vi "Board Calibrator.vi"(7 "Board":T1 items=["Quad DC Board", "Lens 1 (Slot 8) Module", "Lens 2 (Slot 6) Module", "Detector Board", "Quad DC Board with Test Points", "Lens 1 Module with Test Points", "Len 2 Module with Test Points", "", "", "", "", "", "", "", ""]) -> (2 "ADC Table":T2[](array[typedef]), 3 "Suceeded":bool)   [LabVIEW 2018]
uses:
  Type/_RT Configuration 2.ctl
  Type/_Board ID.ctl
  Type/_Model Family.ctl
  Type/_RT Command.ctl
  <vilib>/printing/EasyPrintingControls.llb/layout_options.ctl
  <vilib>/printing/EasyPrintingControls.llb/orientation.ctl
  <vilib>/printing/EasyPrintingControls.llb/panel_scaling_for_page.ctl
  <vilib>/printing/EasyPrintingControls.llb/margins.ctl
  <vilib>/printing/EasyPrintingControls.llb/margin_values.ctl
  <vilib>/printing/EasyPrintingControls.llb/measurement_system.ctl
  <vilib>/printing/EasyPrintingControls.llb/printer_options.ctl
  <vilib>/printing/EasyPrintingControls.llb/printing_method.ctl
  <vilib>/printing/EasyPrintingControls.llb/color_or_monochrome.ctl
  <vilib>/printing/EasyPrintingControls.llb/page_header_options.ctl
  <vilib>/printing/EasyPrintingControls.llb/page_headers.ctl
  <vilib>/printing/EasyPrintingControls.llb/page_header_content_options.ctl
  <vilib>/printing/EasyPrinting.llb/Easy Print VI Panel or Documentation (path).vi
  <vilib>/Utility/NIReport.llb/NI_ReportGenerationCore.lvlib
panel:
  in  "Print":bool
  in  "ADC Channel Calibration":string[][](table)
  in  "Done":bool
  in  "Start":bool
  in  "DAC Channel Calibration":string[][](table)
  out "Current Task":string="Press Start Calibration button to begin or Done button to exit"
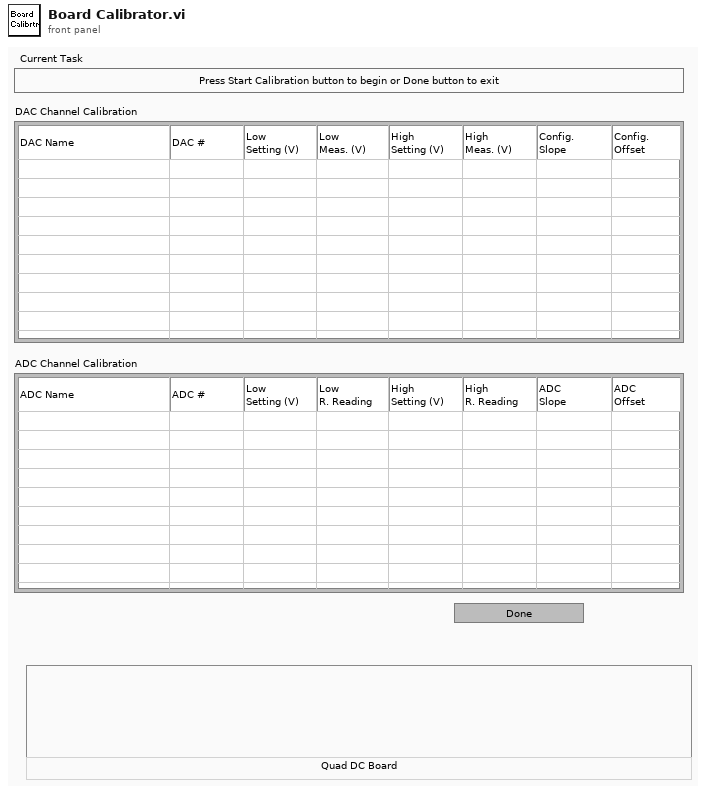
[diagram p1: front panel]
types:
  T1 = typedef "_Board ID.ctl" = u16
  T2 = typedef "_RT Configuration 2.ctl" = cluster{"Name":string, "Ch#":u8, "Min":dbl, "Max":dbl, "Def+":dbl, "Def-":dbl, "Offset":dbl, "Slope":dbl, "Type":u8, "Description":string, "SettleT":dbl}
  T3 = typedef "_RT Command.ctl" = enum16{"xml Start Run", "xml Start Actual Run", "xml Stop Run", "xml Runtime Update", "xml Get Status", "xml Get Table", "xml Set Table", "xml Get Configuration", "xml System Status", "xml Set LC Input Logic", "xml Get Data", "xml Get Info", "Start", "StartActualRun", "Stop", "Runtime Update", "Get Data", "Get Info", "Get Status", "Get Param", "Get Config", "Get Table", "Read ADC", "Set Oscillator", "Update Config", "Update Table", "Set All Pol", "Set Pol and DC", "Set Max Mass", "Toggle RP", "Toggle EL", "Set PIC", "Initialize Turbo", "Send Turbo Comm", "Close Turbo", "P1", "P2", "P3", "Send Serial", "Set LC Out", "Get LC In", "Read VAC", "Test Table", "Toggle Power", "Get Startup", "Set Startup", "Get ADC Table", "Set ADC Table", "Get Brief Status", "Get Detail Status", "Auxiliary Update", "Set CC Logics", "Test Channel", "Set CC Input Logics", "Ignore Error", "invalid"}
  T4 = typedef "NI_ReportGenerationCore.lvlib/layout_options.ctl" = cluster{"orientation (unchanged)":T5, "panel scaling for page (unchanged)":T6, "margins":T7, "printer options":T10, "page header options":T13}
  T5 = typedef "NI_ReportGenerationCore.lvlib/orientation.ctl" = u16
  T6 = typedef "NI_ReportGenerationCore.lvlib/panel_scaling_for_page.ctl" = u16
  T7 = typedef "NI_ReportGenerationCore.lvlib/margins.ctl" = cluster{"override VI margins (false)":bool, "margins (1.00)":T8, "measurement system (default)":T9}
  T8 = typedef "NI_ReportGenerationCore.lvlib/margin_values.ctl" = cluster{"top":dbl, "left":dbl, "right":dbl, "bottom":dbl}
  T9 = typedef "NI_ReportGenerationCore.lvlib/measurement_system.ctl" = u16
  T10 = typedef "NI_ReportGenerationCore.lvlib/printer_options.ctl" = cluster{"destination printer name (current)":string, "printing method (unchanged)":T11, "color or monochrome (unchanged)":T12}
  T11 = typedef "NI_ReportGenerationCore.lvlib/printing_method.ctl" = u16
  T12 = typedef "NI_ReportGenerationCore.lvlib/color_or_monochrome.ctl" = u16
  T13 = typedef "NI_ReportGenerationCore.lvlib/page_header_options.ctl" = cluster{"page headers (unchanged)":T14, "page header content options":T15}
  T14 = typedef "NI_ReportGenerationCore.lvlib/page_headers.ctl" = u16
  T15 = typedef "NI_ReportGenerationCore.lvlib/page_header_content_options.ctl" = cluster{"Include VI Name":bool, "Include VI Path":bool, "Include Last Modification Date":bool, "Include Date Printed":bool, "Include Page Number":bool, "Include VI Icon":bool}
  T16 = typedef "_Model Family.ctl" = u16
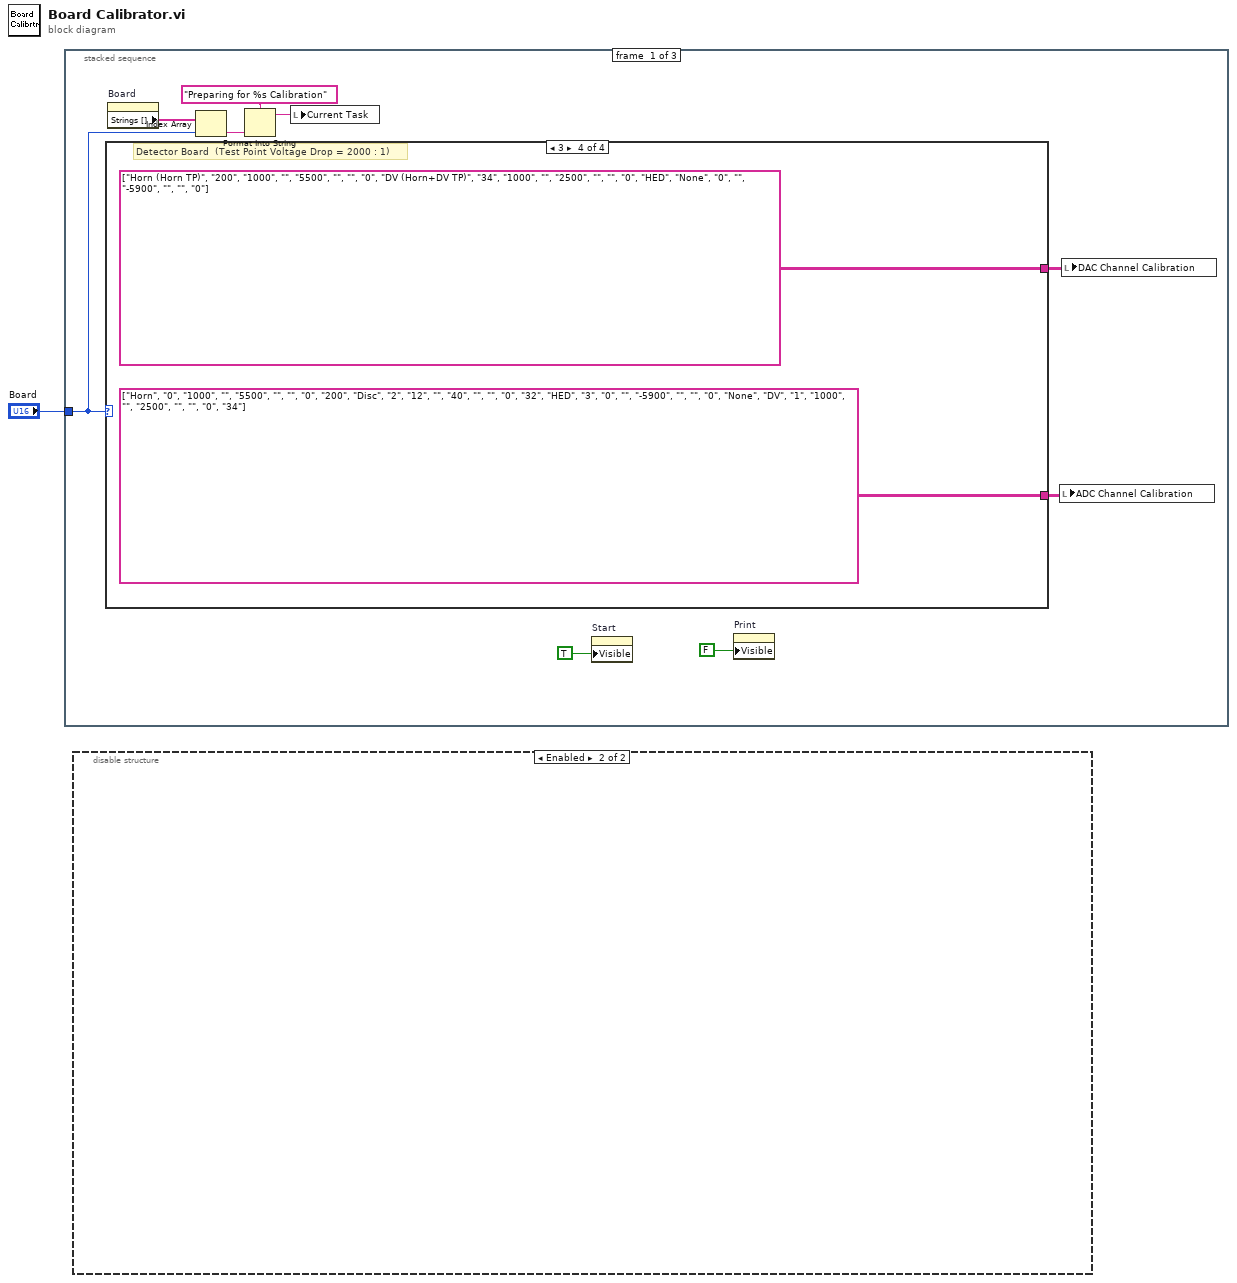
[diagram p0: block diagram]
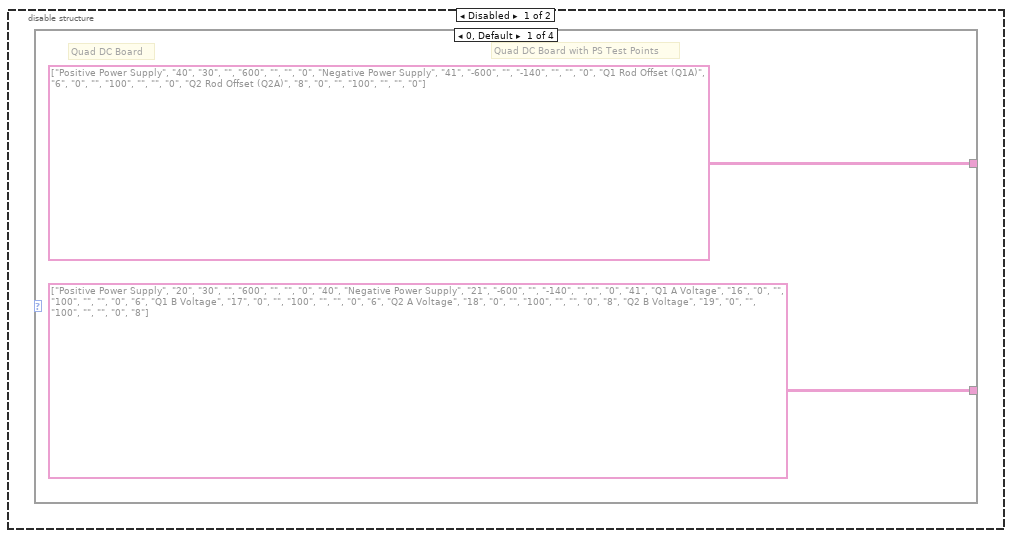
[diagram p2: hidden frame]
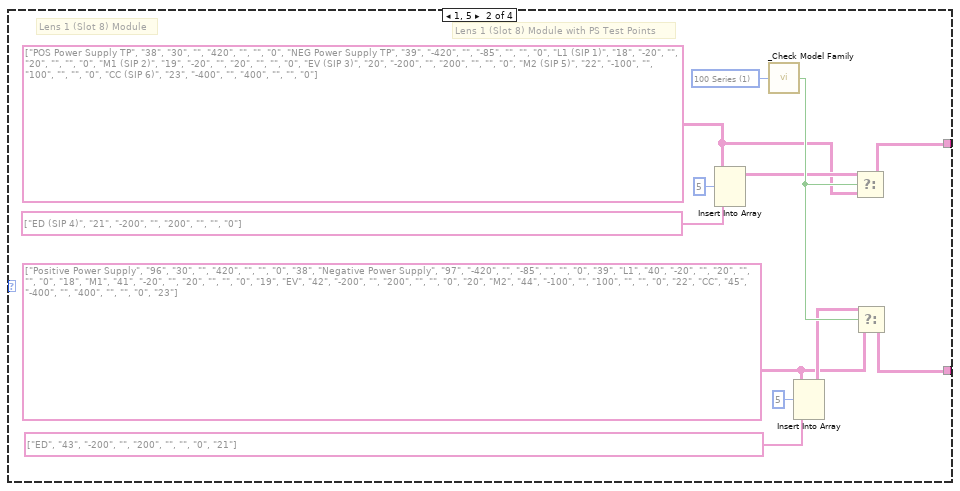
[diagram p3: hidden frame]
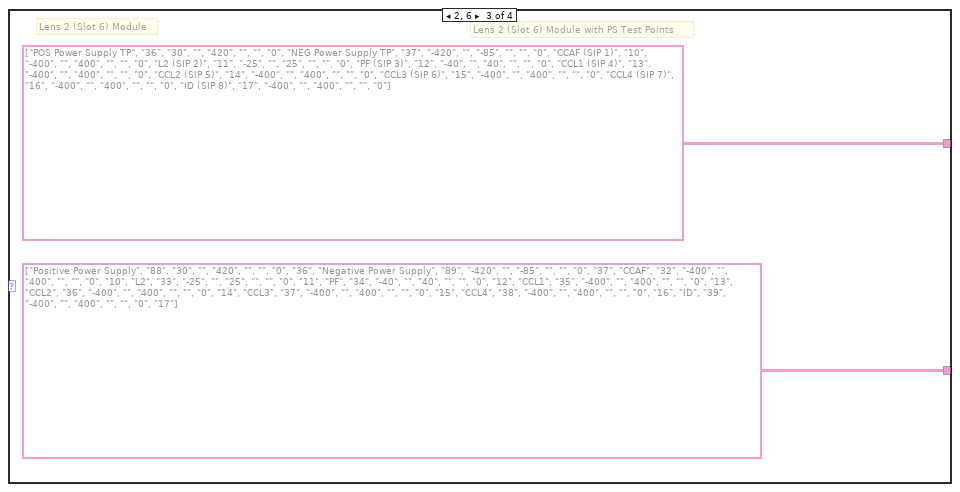
[diagram p4: hidden frame]
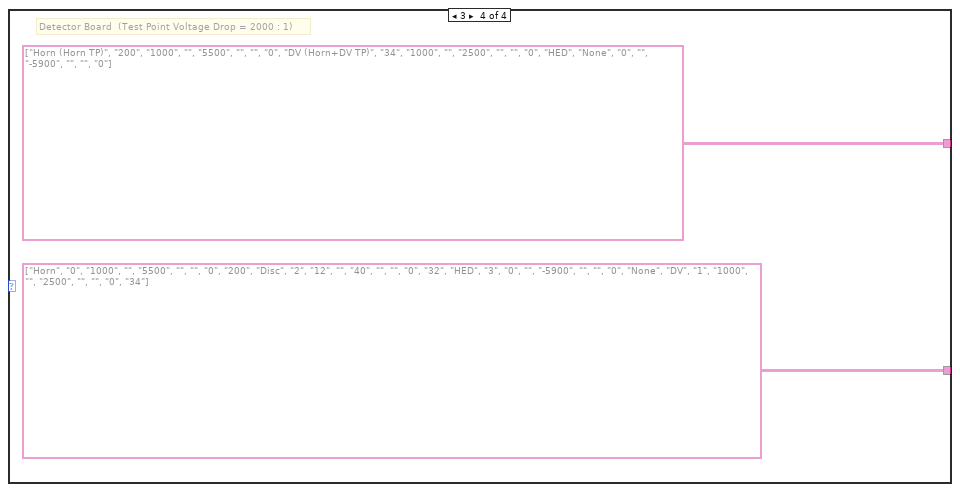
[diagram p5: hidden frame]
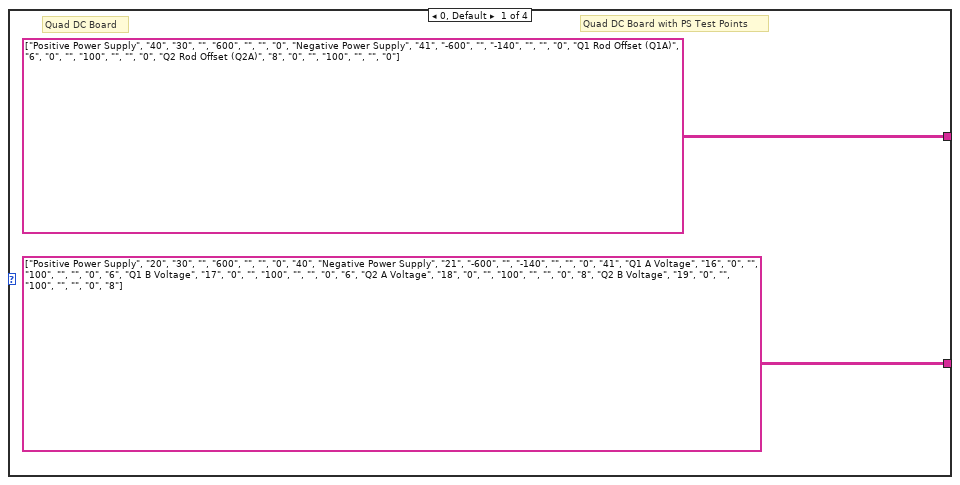
[diagram p6: hidden frame]
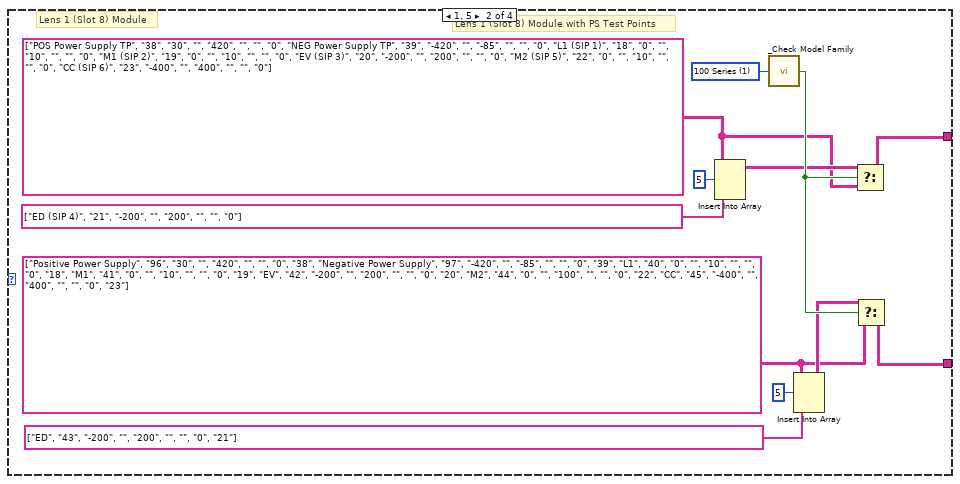
[diagram p7: hidden frame]
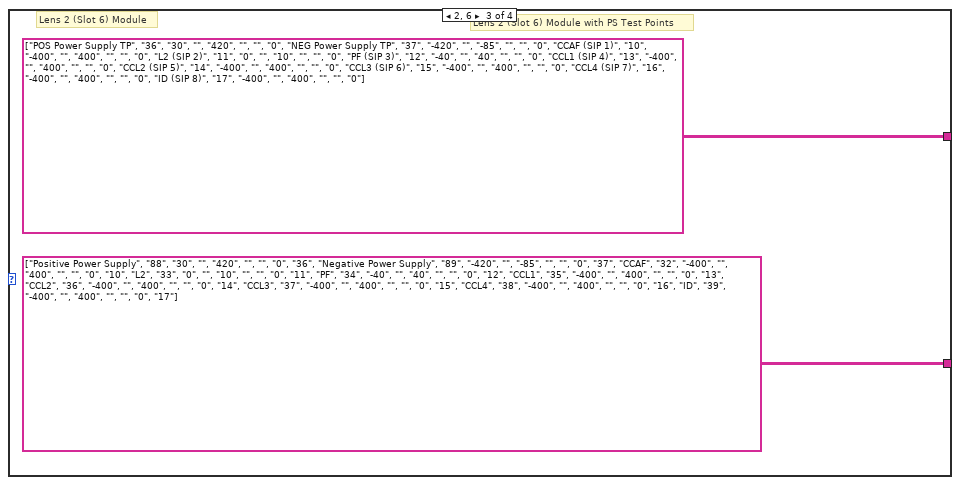
[diagram p8: hidden frame]
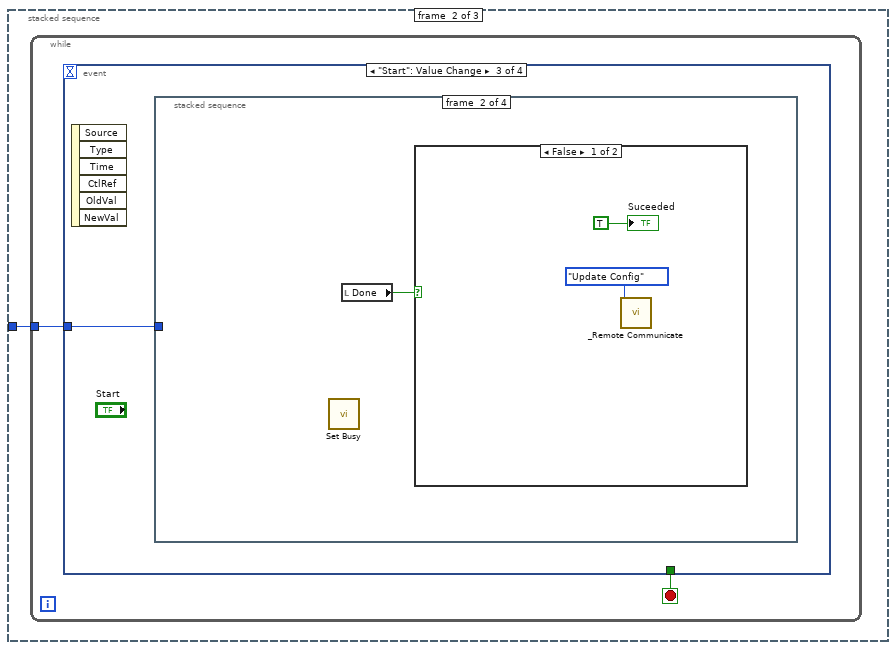
[diagram p9: hidden frame]
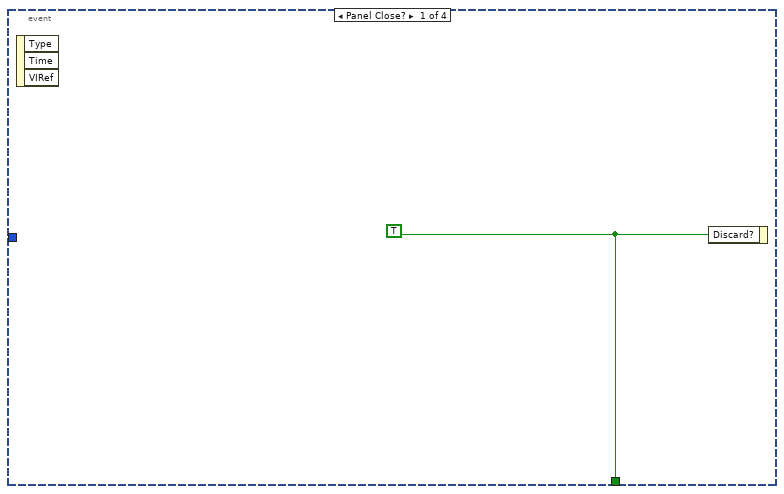
[diagram p10: hidden frame]
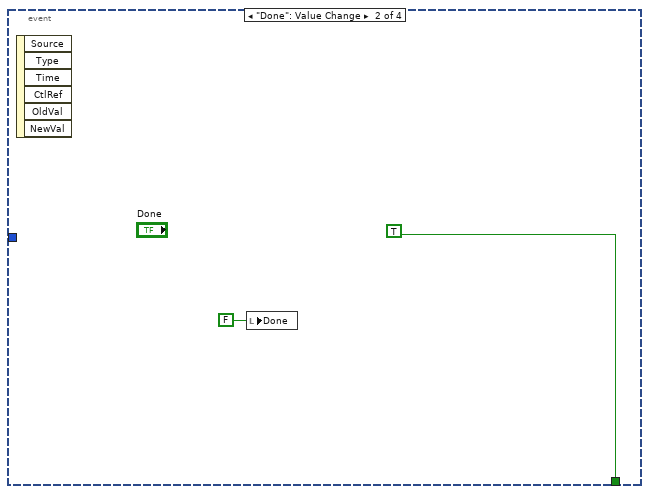
[diagram p11: hidden frame]
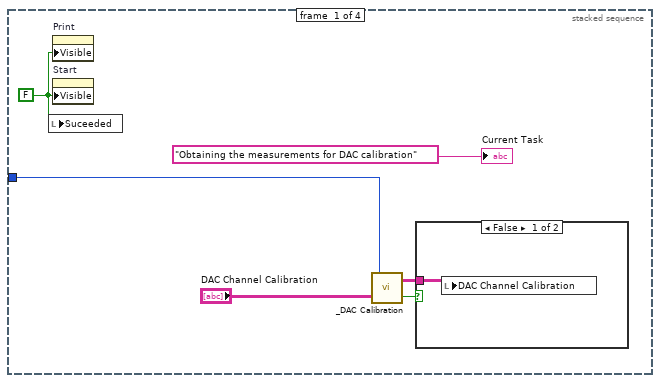
[diagram p12: hidden frame]
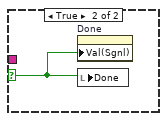
[diagram p13: hidden frame]
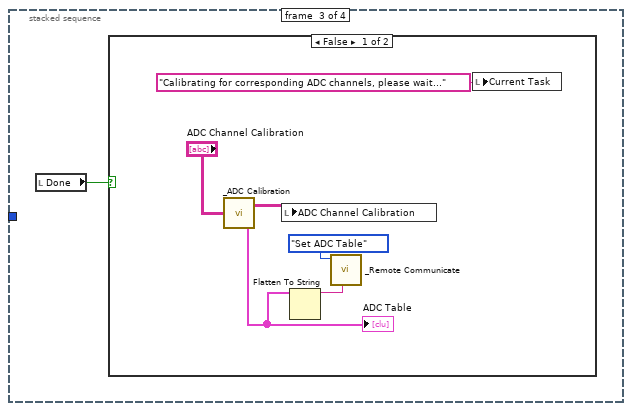
[diagram p15: hidden frame]
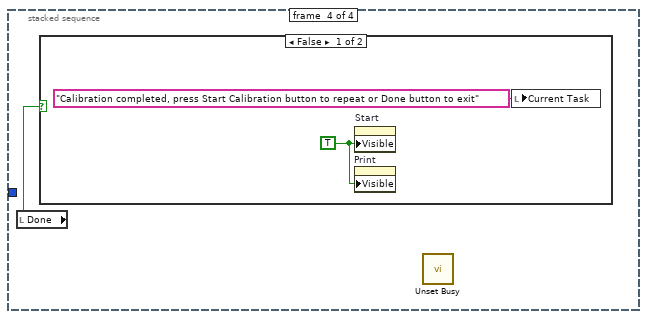
[diagram p17: hidden frame]
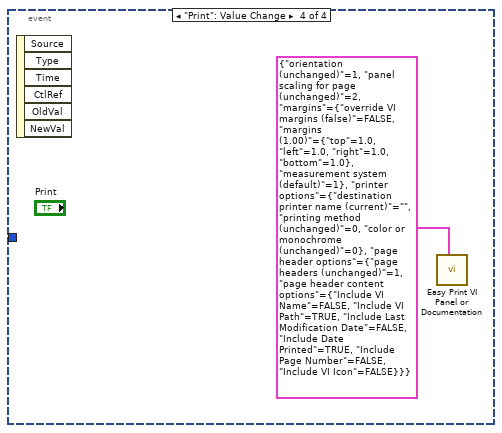
[diagram p19: hidden frame]
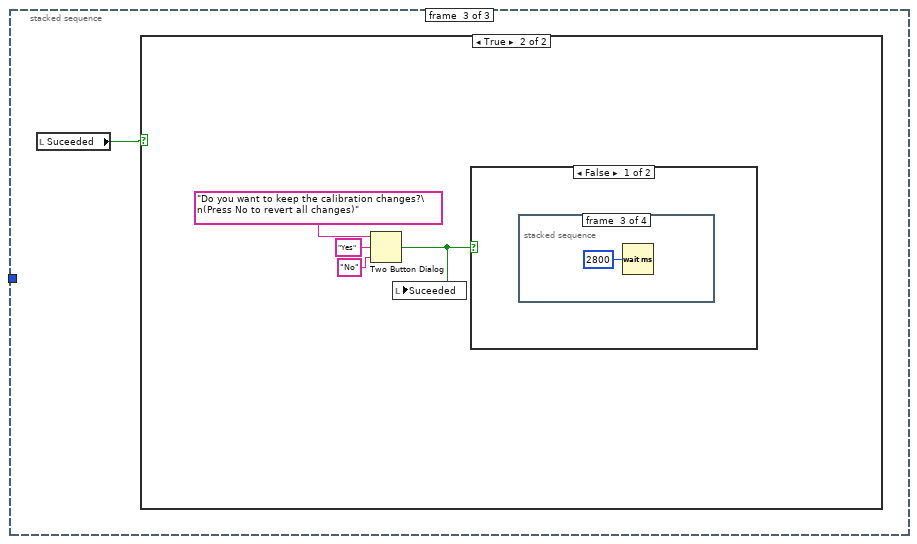
[diagram p20: hidden frame]
diagram:
  n1 = stacked-sequence {
    tunnel: "Board" -> [w6 w29 _]
    frame #0 {
      n2 = case shown="3" w6 {
        tunnel: [string[][] [["Positive Power Supply", "20", "30", "", "600", "", "", "0", "40"], ["Negative Power Supply", "21", "-600", "", "-140", "", "", "0", "41"], ["Q1 A Voltage", "16", "0", "", "100", "", "", "0", "6"], ["Q1 B Voltage", "17", "0", "", "100", "", "", "0", "6"], ["Q2 A Voltage", "18", "0", "", "100", "", "", "0", "8"], ["Q2 B Voltage", "19", "0", "", "100", "", "", "0", "8"]] ("ADC Channel Calibration") w13 string[][] [["Positive Power Supply", "88", "30", "", "420", "", "", "0", "36"], ["Negative Power Supply", "89", "-420", "", "-85", "", "", "0", "37"], ["CCAF", "32", "-400", "", "400", "", "", "0", "10"], ["L2", "33", "0", "", "10", "", "", "0", "11"], ["PF", "34", "-40", "", "40", "", "", "0", "12"], ["CCL1", "35", "-400", "", "400", "", "", "0", "13"], ["CCL2", "36", "-400", "", "400", "", "", "0", "14"], ["CCL3", "37", "-400", "", "400", "", "", "0", "15"], ["CCL4", "38", "-400", "", "400", "", "", "0", "16"], ["ID", "39", "-400", "", "400", "", "", "0", "17"]] ("ADC Channel Calibration") string[][] [["Horn", "0", "1000", "", "5500", "", "", "0", "200"], ["Disc", "2", "12", "", "40", "", "", "0", "32"], ["HED", "3", "0", "", "-5900", "", "", "0", "None"], ["DV", "1", "1000", "", "2500", "", "", "0", "34"]] ("ADC Channel Calibration")] -> w10
        tunnel: [string[][] [["Positive Power Supply", "40", "30", "", "600", "", "", "0"], ["Negative Power Supply", "41", "-600", "", "-140", "", "", "0"], ["Q1 Rod Offset (Q1A)", "6", "0", "", "100", "", "", "0"], ["Q2 Rod Offset (Q2A)", "8", "0", "", "100", "", "", "0"]] ("DAC Channel Calibration") w16 string[][] [["POS Power Supply TP", "36", "30", "", "420", "", "", "0"], ["NEG Power Supply TP", "37", "-420", "", "-85", "", "", "0"], ["CCAF (SIP 1)", "10", "-400", "", "400", "", "", "0"], ["L2 (SIP 2)", "11", "0", "", "10", "", "", "0"], ["PF (SIP 3)", "12", "-40", "", "40", "", "", "0"], ["CCL1 (SIP 4)", "13", "-400", "", "400", "", "", "0"], ["CCL2 (SIP 5)", "14", "-400", "", "400", "", "", "0"], ["CCL3 (SIP 6)", "15", "-400", "", "400", "", "", "0"], ["CCL4 (SIP 7)", "16", "-400", "", "400", "", "", "0"], ["ID (SIP 8)", "17", "-400", "", "400", "", "", "0"]] ("DAC Channel Calibration") string[][] [["Horn (Horn TP)", "200", "1000", "", "5500", "", "", "0"], ["DV (Horn+DV TP)", "34", "1000", "", "2500", "", "", "0"], ["HED", "None", "0", "", "-5900", "", "", "0"]] ("DAC Channel Calibration")] -> w9
        frame 0, Default {
          # "Quad DC Board with PS Test Points"
          # "Quad DC Board"
        }
        frame 1, 5 {
          w20 = T16 1 items=["8080 Series", "100 Series", "200 Series", "300 Series", "Other Series"] ("Model Family (100)")
          w14 = string[][] [["Positive Power Supply", "96", "30", "", "420", "", "", "0", "38"], ["Negative Power Supply", "97", "-420", "", "-85", "", "", "0", "39"], ["L1", "40", "0", "", "10", "", "", "0", "18"], ["M1", "41", "0", "", "10", "", "", "0", "19"], ["EV", "42", "-200", "", "200", "", "", "0", "20"], ["M2", "44", "0", "", "100", "", "", "0", "22"], ["CC", "45", "-400", "", "400", "", "", "0", "23"]] ("ADC Channel Calibration")
          w17 = string[][] [["POS Power Supply TP", "38", "30", "", "420", "", "", "0"], ["NEG Power Supply TP", "39", "-420", "", "-85", "", "", "0"], ["L1 (SIP 1)", "18", "0", "", "10", "", "", "0"], ["M1 (SIP 2)", "19", "0", "", "10", "", "", "0"], ["EV (SIP 3)", "20", "-200", "", "200", "", "", "0"], ["M2 (SIP 5)", "22", "0", "", "10", "", "", "0"], ["CC (SIP 6)", "23", "-400", "", "400", "", "", "0"]] ("DAC Channel Calibration")
          # "Lens 1 (Slot 8) Module with PS Test Points"
          # "Lens 1 (Slot 8) Module"
          n3 = Insert Into Array(array=w17, index (row)=5, new element=string[] ["ED (SIP 4)", "21", "-200", "", "200", "", "", "0"] ("new element/subarray")) -> (w18:string[][])  [unwired: 1 in]
          n4 = call "_Check Model Family.vi"("Model Family (100)"=w20) -> ("Yes"=w19:bool)
          n5 = Insert Into Array(array=w14, index (row)=5, new element=string[] ["ED", "43", "-200", "", "200", "", "", "0", "21"] ("new element/subarray")) -> (w15:string[][])  [unwired: 1 in]
          n6 = Select(t=w18, s=w19, f=w17) -> (s? t:f=w16:string[][])
          n7 = Select(t=w15, s=w19, f=w14) -> (s? t:f=w13:string[][])
        }
        frame 2, 6 {
          # "Lens 2 (Slot 6) Module with PS Test Points"
          # "Lens 2 (Slot 6) Module"
        }
        frame 3 {
          # "Detector Board  (Test Point Voltage Drop = 2000 : 1)"
        }
      }
      n8 = property on="Board" class="Ring (strict)"() -> ("Strings []"=w5:string[])  [unwired: 2 in, 2 out]
      n9 = Index Array(array=w5, index=w6) -> (element=w2:string)
      n10 = Format Into String(format string="Preparing for %s Calibration", w2) -> (resulting string=w3:string)  [unwired: 2 in, 1 out]
      n11 = local write "Current Task"(w3) -> ()
      n12 = property on="Start" class="Bool"("Visible"=TRUE) -> ()  [unwired: 2 in, 2 out]
      n13 = property on="Print" class="Bool"("Visible"=FALSE) -> ()  [unwired: 2 in, 2 out]
      n14 = local write "ADC Channel Calibration"(w10) -> ()
      n15 = local write "DAC Channel Calibration"(w9) -> ()
    }
    frame #1 {
      n16 = while {
        tunnel: w29 -> [w30]
        stop <- w31 stop-if-true
        n17 = event shown="[2] \"Start\": Value Change" {
          selector: _ -> [_ _ _ _]
          dyn-events: _ -> [_ _ _ _]
          timeout: _ -> [_ _ _ _]
          tunnel: [w32 TRUE _ _] -> w31
          tunnel: w30 -> [_ _ w35 _]
          event Panel Close? {
            w32 = TRUE
            n18 = event-data() -> ()  [unwired: 4 out]
            n19 = event-data("Discard?"=w32) -> ()  [unwired: 1 in, 1 out]
          }
          event "Done": Value Change {
            n20 = event-data() -> ()  [unwired: 7 out]
            n21 = local write "Done"(FALSE ("Done")) -> ()
          }
          event "Start": Value Change {
            n22 = event-data() -> ()  [unwired: 7 out]
            n23 = stacked-sequence {
              tunnel: w35 -> [w41 _ _ _]
              frame #0 {
                w40 = FALSE ("Visible")
                n24 = local write "Suceeded"(w40) -> ()
                n25 = property on="Print" class="Bool"("Visible"=w40) -> ()  [unwired: 2 in, 2 out]
                n26 = property on="Start" class="Bool"("Visible"=w40) -> ()  [unwired: 2 in, 2 out]
                n27 = call "_DAC Calibration.vi"("DAC in"="DAC Channel Calibration", "Board"=w41) -> ("aborted"=w36:bool, "DAC out"=w37:string[][])
                n28 = case shown="False" w36 {
                  selector: w36 -> [_ w43]
                  tunnel: w37 -> [w42 _]
                  frame False {
                    n29 = local write "DAC Channel Calibration"(w42) -> ()
                  }
                  frame True {
                    n30 = property on="Done" class="Bool (strict)"("Val(Sgnl)"=w43) -> ()  [unwired: 2 in, 2 out]
                    n31 = local write "Done"(w43) -> ()
                  }
                }
                "Current Task" <- "Obtaining the measurements for DAC calibration" ("Current Task")
              }
              frame #1 {
                n32 = call <vilib>:"Set Busy.vi"() -> ()  [unwired: 4 in, 8 out]
                n33 = local read "Done"() -> (w44:bool)
                n34 = case shown="False" w44 {
                  frame False {
                    n35 = call "_Remote Communicate.vi"("Command"=_RT_Command."Update Config") -> ()  [unwired: 5 in, 4 out]
                    "Suceeded" <- TRUE ("Suceeded")
                  }
                  frame True {
                  }
                }
              }
              frame #2 {
                n36 = local read "Done"() -> (w47:bool)
                n37 = case shown="False" w47 {
                  frame False {
                    n38 = call "_ADC Calibration.vi"("ADC In"="ADC Channel Calibration") -> ("ADC Out"=w51:string[][], "ADC Table"=w48:T2[])
                    "ADC Table" <- w48
                    n39 = local write "ADC Channel Calibration"(w51) -> ()
                    n40 = Flatten To String(anything=w48) -> (data string=w49:string)  [unwired: 1 in, 4 out]
                    n41 = call "_Remote Communicate.vi"("String"=w49, "Command"=_RT_Command."Set ADC Table") -> ()  [unwired: 4 in, 4 out]
                    n42 = local write "Current Task"("Calibrating for corresponding ADC channels, please wait..." ("Current Task")) -> ()
                  }
                  frame True {
                  }
                }
              }
              frame #3 {
                n43 = local read "Done"() -> (w54:bool)
                n44 = case shown="False" w54 {
                  frame False {
                    w55 = TRUE ("Visible")
                    n45 = property on="Start" class="Bool"("Visible"=w55) -> ()  [unwired: 2 in, 2 out]
                    n46 = property on="Print" class="Bool"("Visible"=w55) -> ()  [unwired: 2 in, 2 out]
                    n47 = local write "Current Task"("Calibration completed, press Start Calibration button to repeat or Done button to exit" ("Current Task")) -> ()
                  }
                  frame True {
                  }
                }
                n48 = call <vilib>:"Unset Busy.vi"() -> ()  [unwired: 2 in, 10 out]
              }
            }
          }
          event "Print": Value Change {
            n49 = event-data() -> ()  [unwired: 7 out]
            n50 = call-poly <vilib>:"Easy Print VI Panel or Documentation.vi"("layout options"=T4 {"orientation (unchanged)"=1, "panel scaling for page (unchanged)"=2, "margins"={"override VI margins (false)"=FALSE, "margins (1.00)"={"top"=1.0, "left"=1.0, "right"=1.0, "bottom"=1.0}, "measurement system (default)"=1}, "printer options"={"destination printer name (current)"="", "printing method (unchanged)"=0, "color or monochrome (unchanged)"=0}, "page header options"={"page headers (unchanged)"=1, "page header content options"={"Include VI Name"=FALSE, "Include VI Path"=TRUE, "Include Last Modification Date"=FALSE, "Include Date Printed"=TRUE, "Include Page Number"=FALSE, "Include VI Icon"=FALSE}}}) -> ()  [unwired: 4 in, 7 out]
          }
        }
      }
    }
    frame #2 {
      n51 = local read "Suceeded"() -> (w58:bool)
      n52 = case shown="True" w58 {
        frame False {
        }
        frame True {
          n53 = Two Button Dialog(message="Do you want to keep the calibration changes?\n(Press No to revert all changes)" ("format string"), 1:"No" ("F button name (\"Cancel\")"), 2:"Yes" ("T button name (\"OK\")")) -> (T button?=w59:bool)
          n54 = local write "Suceeded"(w59) -> ()
          n55 = case shown="False" w59 {
            frame False {
              n56 = stacked-sequence {
                frame #0 {
                  n57 = call <vilib>:"Set Busy.vi"() -> ()  [unwired: 4 in, 8 out]
                }
                frame #1 {
                  n58 = call "_Load All Tables.vi"("Use temporary file (F)"=TRUE) -> ()  [unwired: 7 out]
                }
                frame #2 {
                  n59 = Wait (ms)(milliseconds to wait=u32 2800) -> ()  [unwired: 1 out]
                }
                frame #3 {
                  n60 = call <vilib>:"Unset Busy.vi"() -> ()  [unwired: 2 in, 10 out]
                }
              }
            }
            frame True {
            }
          }
        }
      }
    }
  }
  n61 = disable-structure shown="Enabled" {
    frame Disabled {
      n62 = case shown="0, Default" {
        selector: _ -> [_ _ _ _]
        tunnel: [string[][] [["Positive Power Supply", "20", "30", "", "600", "", "", "0", "40"], ["Negative Power Supply", "21", "-600", "", "-140", "", "", "0", "41"], ["Q1 A Voltage", "16", "0", "", "100", "", "", "0", "6"], ["Q1 B Voltage", "17", "0", "", "100", "", "", "0", "6"], ["Q2 A Voltage", "18", "0", "", "100", "", "", "0", "8"], ["Q2 B Voltage", "19", "0", "", "100", "", "", "0", "8"]] ("ADC Channel Calibration") w67 string[][] [["Positive Power Supply", "88", "30", "", "420", "", "", "0", "36"], ["Negative Power Supply", "89", "-420", "", "-85", "", "", "0", "37"], ["CCAF", "32", "-400", "", "400", "", "", "0", "10"], ["L2", "33", "-25", "", "25", "", "", "0", "11"], ["PF", "34", "-40", "", "40", "", "", "0", "12"], ["CCL1", "35", "-400", "", "400", "", "", "0", "13"], ["CCL2", "36", "-400", "", "400", "", "", "0", "14"], ["CCL3", "37", "-400", "", "400", "", "", "0", "15"], ["CCL4", "38", "-400", "", "400", "", "", "0", "16"], ["ID", "39", "-400", "", "400", "", "", "0", "17"]] ("ADC Channel Calibration") string[][] [["Horn", "0", "1000", "", "5500", "", "", "0", "200"], ["Disc", "2", "12", "", "40", "", "", "0", "32"], ["HED", "3", "0", "", "-5900", "", "", "0", "None"], ["DV", "1", "1000", "", "2500", "", "", "0", "34"]] ("ADC Channel Calibration")] -> _
        tunnel: [string[][] [["Positive Power Supply", "40", "30", "", "600", "", "", "0"], ["Negative Power Supply", "41", "-600", "", "-140", "", "", "0"], ["Q1 Rod Offset (Q1A)", "6", "0", "", "100", "", "", "0"], ["Q2 Rod Offset (Q2A)", "8", "0", "", "100", "", "", "0"]] ("DAC Channel Calibration") w70 string[][] [["POS Power Supply TP", "36", "30", "", "420", "", "", "0"], ["NEG Power Supply TP", "37", "-420", "", "-85", "", "", "0"], ["CCAF (SIP 1)", "10", "-400", "", "400", "", "", "0"], ["L2 (SIP 2)", "11", "-25", "", "25", "", "", "0"], ["PF (SIP 3)", "12", "-40", "", "40", "", "", "0"], ["CCL1 (SIP 4)", "13", "-400", "", "400", "", "", "0"], ["CCL2 (SIP 5)", "14", "-400", "", "400", "", "", "0"], ["CCL3 (SIP 6)", "15", "-400", "", "400", "", "", "0"], ["CCL4 (SIP 7)", "16", "-400", "", "400", "", "", "0"], ["ID (SIP 8)", "17", "-400", "", "400", "", "", "0"]] ("DAC Channel Calibration") string[][] [["Horn (Horn TP)", "200", "1000", "", "5500", "", "", "0"], ["DV (Horn+DV TP)", "34", "1000", "", "2500", "", "", "0"], ["HED", "None", "0", "", "-5900", "", "", "0"]] ("DAC Channel Calibration")] -> _
        frame 0, Default {
          # "Quad DC Board with PS Test Points"
          # "Quad DC Board"
        }
        frame 1, 5 {
          w74 = T16 1 items=["8080 Series", "100 Series", "200 Series", "300 Series", "Other Series"] ("Model Family (100)")
          w68 = string[][] [["Positive Power Supply", "96", "30", "", "420", "", "", "0", "38"], ["Negative Power Supply", "97", "-420", "", "-85", "", "", "0", "39"], ["L1", "40", "-20", "", "20", "", "", "0", "18"], ["M1", "41", "-20", "", "20", "", "", "0", "19"], ["EV", "42", "-200", "", "200", "", "", "0", "20"], ["M2", "44", "-100", "", "100", "", "", "0", "22"], ["CC", "45", "-400", "", "400", "", "", "0", "23"]] ("ADC Channel Calibration")
          w71 = string[][] [["POS Power Supply TP", "38", "30", "", "420", "", "", "0"], ["NEG Power Supply TP", "39", "-420", "", "-85", "", "", "0"], ["L1 (SIP 1)", "18", "-20", "", "20", "", "", "0"], ["M1 (SIP 2)", "19", "-20", "", "20", "", "", "0"], ["EV (SIP 3)", "20", "-200", "", "200", "", "", "0"], ["M2 (SIP 5)", "22", "-100", "", "100", "", "", "0"], ["CC (SIP 6)", "23", "-400", "", "400", "", "", "0"]] ("DAC Channel Calibration")
          # "Lens 1 (Slot 8) Module with PS Test Points"
          # "Lens 1 (Slot 8) Module"
          n63 = Insert Into Array(array=w71, index (row)=5, new element=string[] ["ED (SIP 4)", "21", "-200", "", "200", "", "", "0"] ("new element/subarray")) -> (w72:string[][])  [unwired: 1 in]
          n64 = call "_Check Model Family.vi"("Model Family (100)"=w74) -> ("Yes"=w73:bool)
          n65 = Insert Into Array(array=w68, index (row)=5, new element=string[] ["ED", "43", "-200", "", "200", "", "", "0", "21"] ("new element/subarray")) -> (w69:string[][])  [unwired: 1 in]
          n66 = Select(t=w72, s=w73, f=w71) -> (s? t:f=w70:string[][])
          n67 = Select(t=w69, s=w73, f=w68) -> (s? t:f=w67:string[][])
        }
        frame 2, 6 {
          # "Lens 2 (Slot 6) Module with PS Test Points"
          # "Lens 2 (Slot 6) Module"
        }
        frame 3 {
          # "Detector Board  (Test Point Voltage Drop = 2000 : 1)"
        }
      }
    }
    frame Enabled {
    }
  }
